vi "ResizeDataArray.vi"(4 "Column":i32, 5 "Row":i32, 6 "Column Max":i32, 7 "Input Array":string[][](array[string])) -> (3 "Output Array":string[][](array[string]))   [LabVIEW 2016]
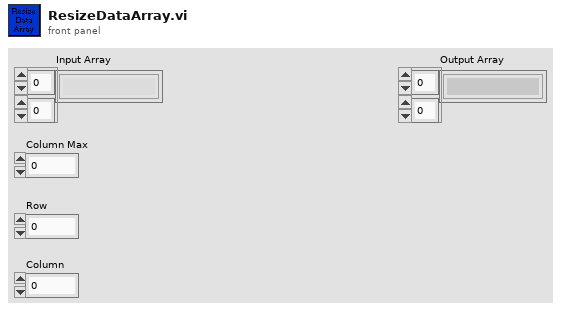
[diagram p1: front panel]
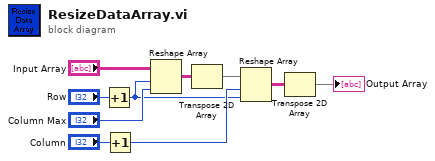
[diagram p0: block diagram]
diagram:
  n1 = Increment(x="Row") -> (x+1=w3:i32)
  n2 = Increment(x="Column") -> (x+1=w4:i32)
  n3 = Reshape Array("Input Array", w3, "Column Max") -> (w6:string[][])
  n4 = Transpose 2D Array(2D array=w6) -> (transposed array=w5:string[][])
  n5 = Reshape Array(w5, w4, w3) -> (w2:string[][])
  n6 = Transpose 2D Array(2D array=w2) -> (transposed array=→"Output Array":string[][])
